vi "save_data.vi"(8 "data 2":cluster{"V":dbl, "dV":dbl, "Q":dbl, "dQ":dbl}[](array[cluster]), 9 "data 1":cluster{"V":dbl, "dV":dbl, "Q":dbl, "dQ":dbl}[](array[cluster]), 10 "times":timestamp[](array[timestamp]), 11 "Filepath":path) -> (0 "error out":errorcluster)   [LabVIEW 2026]
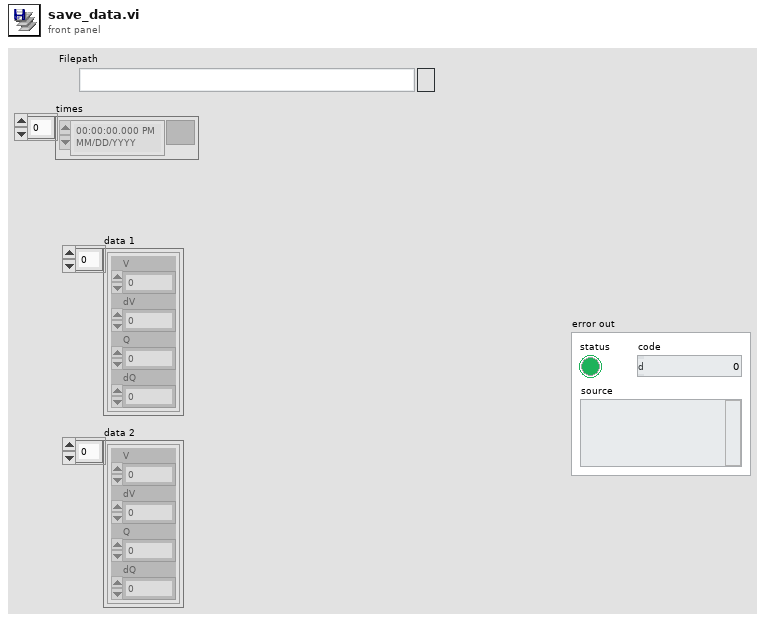
[diagram p1: front panel]
types:
  T1 = enum16{"open", "replace", "create", "open or create", "replace or create", "replace or create with confirmation"}
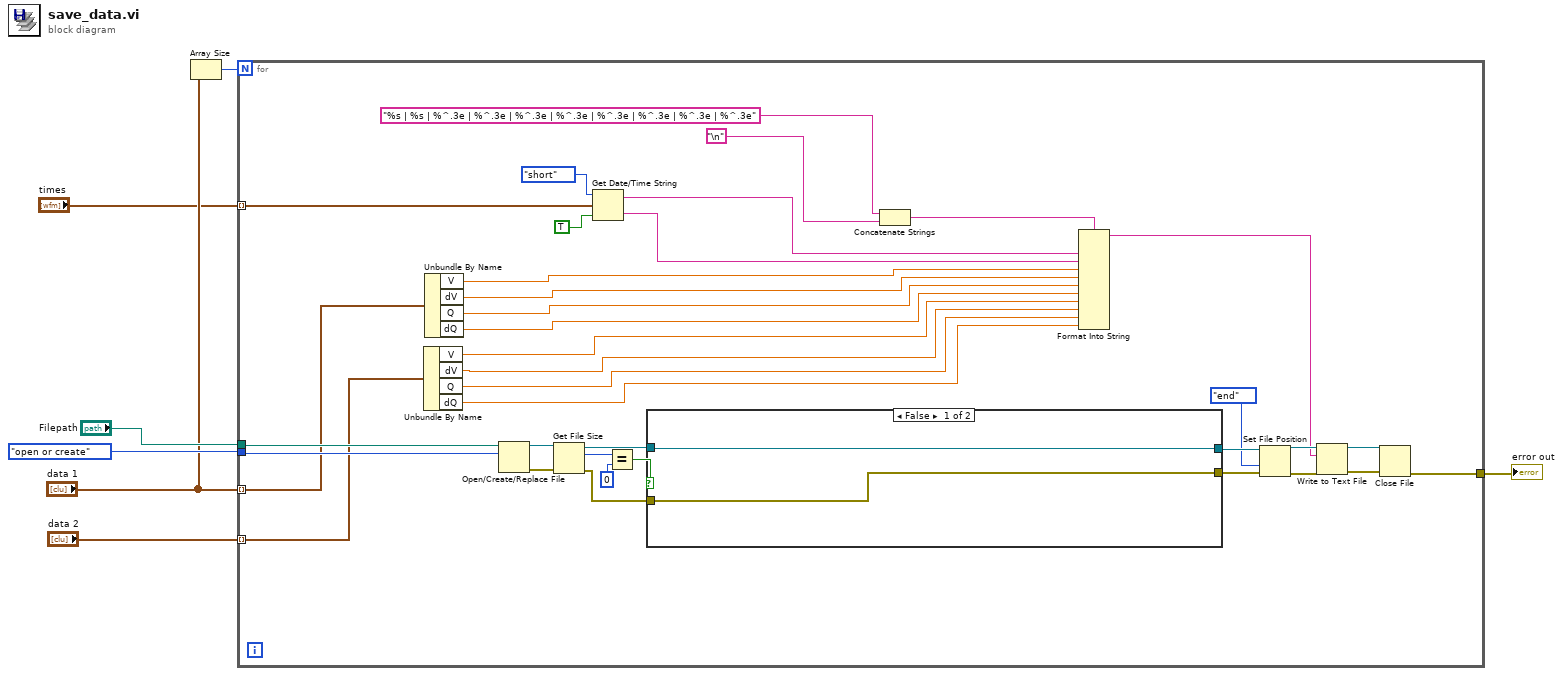
[diagram p0: block diagram]
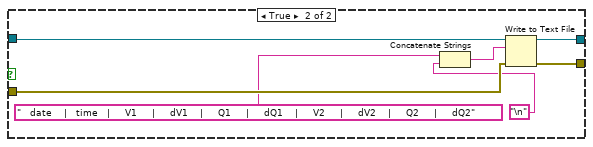
[diagram p2: hidden frame]
diagram:
  n1 = Array Size(array="data 1") -> (size(s)=w4:i32)
  n2 = for {
    N: w4 -> [_]
    tunnel: T1."open or create" ("operation (0:open)") -> [w43]
    tunnel: "Filepath" -> [w26]
    tunnel: "data 1" -> [w25] mode=indexing
    tunnel: "data 2" -> [w20] mode=indexing
    tunnel: [w13] -> w2
    tunnel: "times" -> [w8] mode=indexing
    n3 = Unbundle By Name(w20) -> ("V"=w19:dbl, "dV"=w18:dbl, "Q"=w17:dbl, "dQ"=w16:dbl)
    n4 = Unbundle By Name(w25) -> ("V"=w24:dbl, "dV"=w23:dbl, "Q"=w22:dbl, "dQ"=w21:dbl)
    n5 = Open/Create/Replace File(file path (use dialog)=w26, operation (0:open)=w43) -> (refnum out=w41:refnum<file>, error out=w42:errorcluster)  [unwired: 4 in, 1 out]
    n6 = Get File Size(file=w41, error in=w42) -> (refnum out=w37:refnum<file>, size (in bytes)=w40:i64, 0:w36:errorcluster)
    n7 = Get Date/Time String(date format (0)=enum16{"short", "long", "abbreviated"}."short", seconds (now)=w8, want seconds? (F)=TRUE) -> (date string=w10:string, time string=w9:string)
    n8 = Equal?(x=w40, y=i64 0) -> (x = y?=w38:bool)
    n9 = case shown="False" w38 {
      tunnel: w37 -> [w45 w52]
      tunnel: w36 -> [w44 w51]
      tunnel: [w45 w50] -> w32
      tunnel: [w44 w49] -> w31
      frame False {
      }
      frame True {
        n10 = Concatenate Strings("   date    |   time   |     V1     |     dV1    |     Q1     |     dQ1    |     V2     |     dV2    |     Q2     |     dQ2" ("text"), "\n") -> (w46:string)
        n11 = Write to Text File(file (use dialog)=w52, text=w46, error in=w51) -> (refnum out=w50:refnum<file>, error out=w49:errorcluster)  [unwired: 1 in, 1 out]
      }
    }
    n12 = Concatenate Strings("%s | %s | %^.3e | %^.3e | %^.3e | %^.3e | %^.3e | %^.3e | %^.3e | %^.3e" ("format string"), "\n") -> (w33:string)
    n13 = Format Into String(format string=w33, w10, w9, w24, w23, w22, w21, w19, w18, w17, w16) -> (resulting string=w27:string)  [unwired: 2 in, 1 out]
    n14 = Set File Position(refnum=w32, from (0:start)=enum16{"start", "end", "current"}."end", error in=w31) -> (refnum out=w28:refnum<file>, error out=w29:errorcluster)  [unwired: 1 in]
    n15 = Write to Text File(file (use dialog)=w28, text=w27, error in=w29) -> (refnum out=w14:refnum<file>, error out=w15:errorcluster)  [unwired: 1 in, 1 out]
    n16 = Close File(refnum=w14, error in=w15) -> (error out=w13:errorcluster)  [unwired: 1 out]
  }
  "error out" <- w2
